vi "Dialog_Arrow Key Handler.vi"(10 "String Ref":refnum<vi>, 11 "Tree Ref":refnum<vi>) -> ()   [LabVIEW 2023]
doc: "Called asynchronously, this VI sets the default string (default=\"Filter...\") and the secondary color to the control's text color (default = gray), then monitors the control for a change in focus. When control gains focus, it removes the default string and sets the text to the main text color. When it loses focus, and if string is empty, it sets the value to the default and sets secondary text color.\n\nMake key focus will place the cursor before the default text and handle removing default text if user types any ascii character"
panel:
  in  "Tree":string[](tree)
  in  "Debug String":string
  # "Debug controls:"
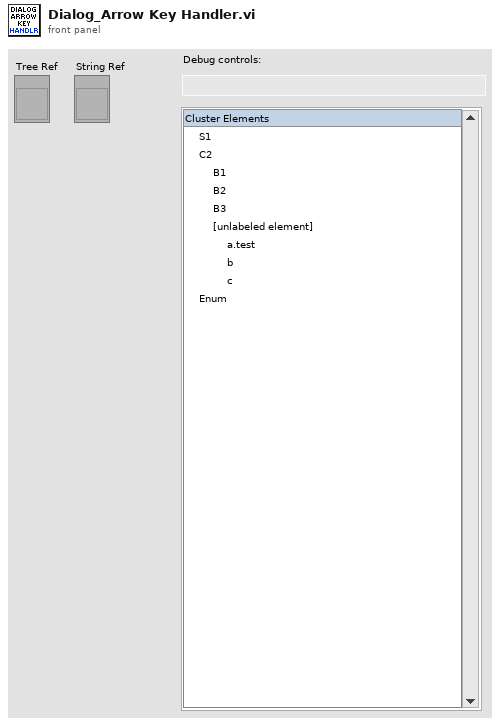
[diagram p1: front panel]
types:
  T1 = typedef "eventvkey.ctl" = enum16{"ASCII", "Enter", "Return", "Shift", "Ctrl", "Alt", "Cmd", "Opt", "Caps", "NumLock", "Clear", "Break", "Up", "Down", "Left", "Right", "Insert", "Delete", "Home", "End", "PageUp", "PageDown", "Escape", "Help", "Pause", "ScrollLock", "F1", "F2", "F3", "F4", "F5", "F6", "F7", "F8", "F9", "F10", "F11", "F12", "F13", "F14", "F15", "F16", "F17", "F18", "F19", "F20", "F21", "F22", "F23", "F24", "Play", "VolumeUp", "VolumeDown", "Mute", "Two Byte Char"}
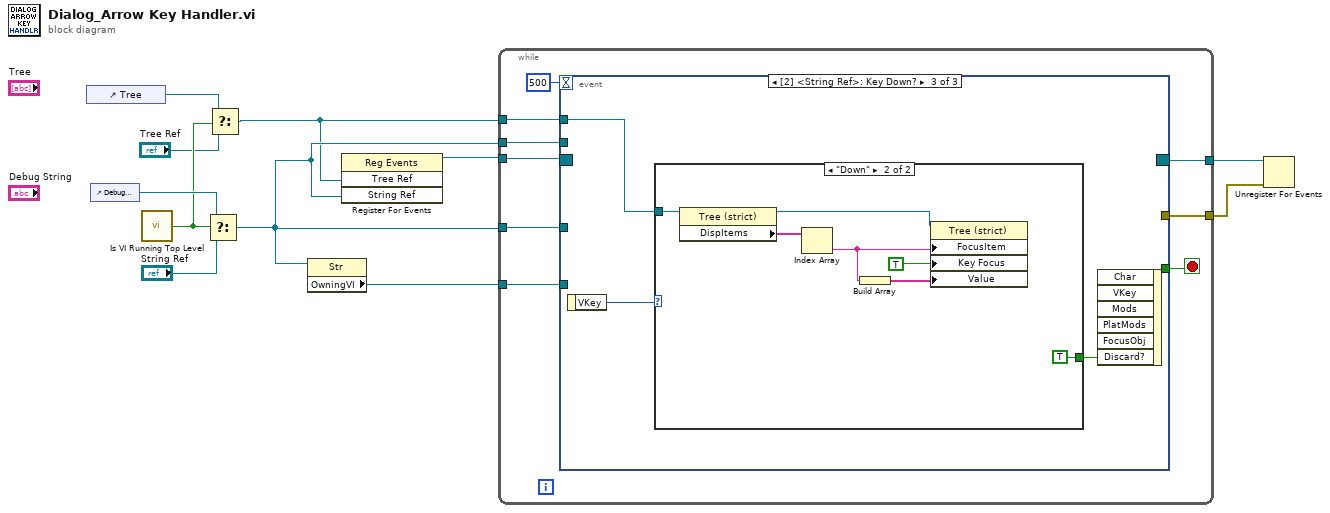
[diagram p0: block diagram]
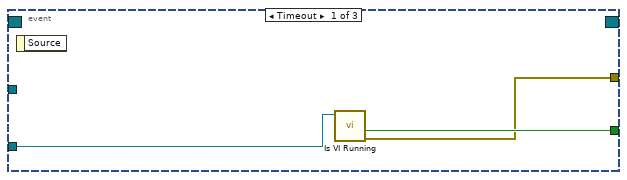
[diagram p2: hidden frame]
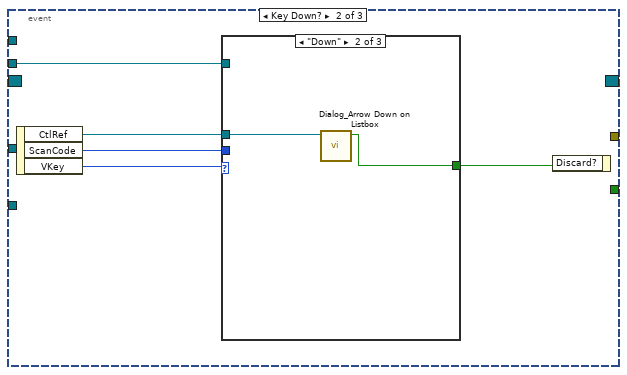
[diagram p3: hidden frame]
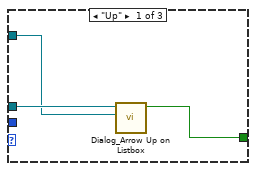
[diagram p4: hidden frame]
diagram:
  n1 = control-ref of="Tree"() -> (w7:refnum<vi>)
  n2 = control-ref of="Debug String"() -> (w11:refnum<vi>)
  n3 = call "Is VI Running Top Level.vi"() -> ("Top Level?"=w9:bool)  [unwired: 5 in]
  n4 = Select(t=w11, s=w9, f="String Ref") -> (s? t:f=w3:refnum<vi>)
  n5 = Select(t=w7, s=w9, f="Tree Ref") -> (s? t:f=w1:refnum<vi>)
  n6 = property class="Str"(reference=w3) -> ("OwningVI"=w2:refnum<vi>)  [unwired: 1 in, 2 out]
  n7 = register-events(w1, w3) -> (reference out=w6:refnum<event-registration>)  [unwired: 2 in, 1 out]
  n8 = while {
    tunnel: w6 -> [w18]
    tunnel: [w17] -> w4
    tunnel: w3 -> [w16]
    tunnel: [w15] -> w5
    tunnel: w3 -> [w14]
    tunnel: w2 -> [w13]
    tunnel: w1 -> [w12]
    stop <- w20 stop-if-true
    n9 = event shown="[2] <String Ref>: Key Down?" {
      selector: w18 -> [_ _ _]
      dyn-events: [_ _ _] -> w15
      timeout: 500 -> [_ _ _]
      tunnel: [w23 _ _] -> w20
      tunnel: [w22 _ _] -> w17
      tunnel: w16 -> [_ _ _]
      tunnel: w14 -> [_ w24 _]
      tunnel: w13 -> [w21 _ _]
      tunnel: w12 -> [_ _ w36]
      event Timeout {
        n10 = event-data() -> ()  [unwired: 1 in, 1 out]
        n11 = call "Is VI Running.vi"("VI in"=w21) -> ("error out"=w22:errorcluster, "VI Not Running"=w23:bool)  [unwired: 7 in, 2 out]
      }
      event Key Down? {
        n12 = event-data() -> ("CtlRef"=w26:refnum<vi>, "ScanCode"=w28:i16, "VKey"=w27:T1)  [unwired: 1 in]
        n13 = case shown="\"Down\"" w27 {
          tunnel: w28 -> [_ _ _]
          tunnel: w26 -> [w31 w33 _]
          tunnel: [w29 w32 _] -> w25
          tunnel: w24 -> [w30 _ _]
          frame "Up" {
            n14 = call "Dialog_Arrow Up on Listbox.vi"("String Ref"=w30, "TreeControl in"=w31) -> ("discard"=w29:bool)  [unwired: 9 in]
          }
          frame "Down" {
            n15 = call "Dialog_Arrow Down on Listbox.vi"("TreeControl in"=w33) -> ("discard"=w32:bool)  [unwired: 10 in]
          }
          frame Default {
          }
        }
        n16 = event-data("Discard?"=w25) -> ()  [unwired: 1 in, 1 out]
      }
      event Key Down? {
        n17 = event-data() -> ("VKey"=w34:T1)  [unwired: 1 in]
        n18 = case shown="\"Down\"" w34 {
          tunnel: w36 -> [_ w43]
          tunnel: [_ TRUE ("Discard?")] -> w35
          frame Default {
          }
          frame "Down" {
            n19 = property class="Tree (strict)"(reference=w43) -> (reference out=w41:refnum<vi>, "DispItems"=w42:string[])  [unwired: 1 in, 1 out]
            n20 = Index Array(array=w42) -> (element=w39:string)  [unwired: 1 in]
            n21 = Build Array(w39) -> (w38:string[])
            n22 = property class="Tree (strict)"(reference=w41, "FocusItem"=w39, "Key Focus"=TRUE, "Value"=w38) -> ()  [unwired: 1 in, 2 out]
          }
        }
        n23 = event-data("Discard?"=w35) -> ()  [unwired: 6 in, 1 out]
      }
    }
  }
  n24 = Unregister For Events(event registration refnum=w5, error in=w4) -> ()  [unwired: 1 out]
